vi "Get Pin Status.vi"(8 "error in (no error)":errorcluster, 9 "Pin":dbl, 10 "Port":dbl, 11 "Simulado in":refnum<class "Simulado.lvclass">) -> (0 "error out":errorcluster, 3 "Simulado out":refnum<class "Simulado.lvclass">)   [LabVIEW 2020, in "Simulado.lvclass"]
doc: "Método heredado del padre con un override"
uses:
  Simulado.lvclass
  Simulado.lvclass/Simulado.ctl
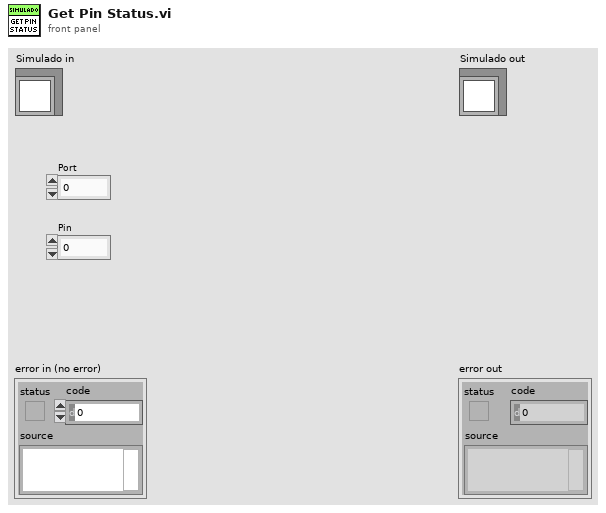
[diagram p1: front panel]
types:
  T1 = typedef "Serial device.lvclass/Brand combobox.ctl" = string
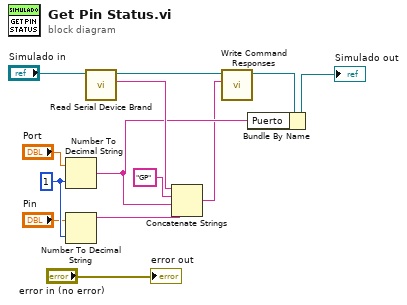
[diagram p0: block diagram]
diagram:
  w10 = i16 1 ("width (-)")
  n1 = Number To Decimal String(number="Port", width (-)=w10) -> (decimal integer string=w2:string)
  n2 = Number To Decimal String(number="Pin", width (-)=w10) -> (decimal integer string=w4:string)
  n3 = call-dynamic "Read Serial Device Brand.vi"("Serial device in"="Simulado in") -> ("Serial Device Brand"=w6:T1, "Serial device out"=w12:refnum<class "Simulado.lvclass">)  [unwired: 8 in, 1 out]
  n4 = Concatenate Strings(w6, "GP" ("string"), w2, w4) -> (w1:string)
  n5 = call-dynamic "Write Command Responses.vi"("Command Responses"=w1, "Simulado in"=w12) -> ("Simulado out"=w11:refnum<class "Simulado.lvclass">)  [unwired: 8 in, 1 out]
  n6 = Bundle By Name(cluster=w11, "Puerto"=w2) -> (→"Simulado out":refnum<class "Simulado.lvclass">)
  "error out" <- "error in (no error)"
